vi "SMO.Activity.GetActivityManager.vi"(8 "error in (no error)":errorcluster, 11 "SMO.Activity":refnum<class "SMO.Activity.lvclass">) -> (0 "error out":errorcluster, 3 "SMO.Activity out":refnum<class "SMO.Activity.lvclass">)   [LabVIEW 2015, in "SMO.Activity.lvclass"]
uses:
  SMO.Activity.lvclass
  SMO.Activity.lvclass/SMO.Activity.ctl
panel:
  # "For instructions on how to use the JKI State Machine Objects, examples and video tutorials, visit:\nhttp://jki.net/state-machine-objects/\n\nJKI State Machine Objects™\nhttp://jki.net/state-machine-objects/\nCopyright (C) 2005-2015, JKI <info@jki.net>\nALL RIGHTS RESERVED"
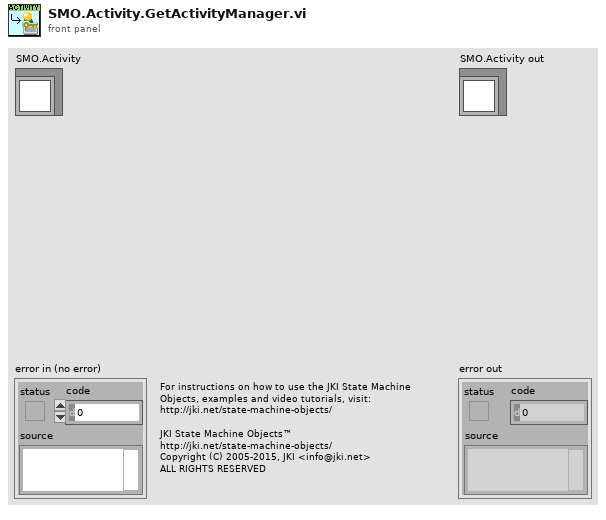
[diagram p1: front panel]
types:
  T1 = typedef "SMO.Activity.lvclass/PrivateData--Ref.ctl" = refnum<data-value>
  T2 = typedef "SMO.Activity.lvclass/PrivateData--Cluster.ctl" = cluster{"Public Events":T3, "Subpanel Ref":refnum<vi>, "UI State":T4}
  T3 = typedef "SMO.Activity.lvclass/PublicEvents--Cluster.ctl" = cluster{"UI State":refnum<user-event>}
  T4 = typedef "SMO.Activity.lvclass/SMO.UI_Embed State--enum.ctl" = enum16{"unknown", "Opened", "Embedded", "Closed"}
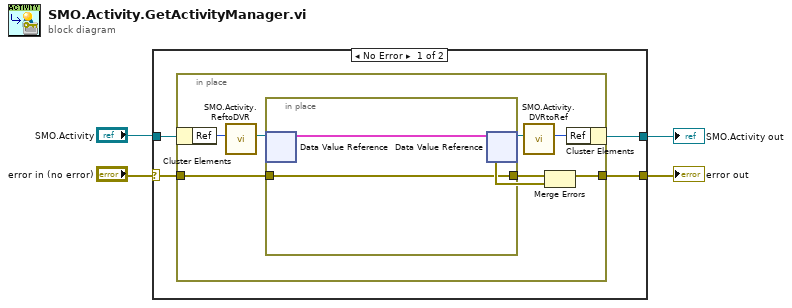
[diagram p0: block diagram]
diagram:
  n1 = case shown="No Error" "error in (no error)" {
    selector: "error in (no error)" -> [w7 w20]
    tunnel: [w6 w20] -> w1
    tunnel: [w5 w19] -> w3
    tunnel: "SMO.Activity" -> [w8 w19]
    frame No Error {
      n2 = in-place {
        in-place-border: w7 -> [w16]
        in-place-border: [w13] -> w6
        n3 = in-place-cluster #1(w8) -> ("Ref"=w10:u32)
        n4 = call "SMO.Activity.ReftoDVR.vi"("Ref"=w10) -> ("Ref"=w9:T1)  [unwired: 10 in]
        n5 = in-place {
          in-place-border: w16 -> [w18]
          in-place-border: [w18] -> w14
          n6 = in-place-dvr #2(w9) -> (w17:T2)  [unwired: 1 out]
          n7 = in-place-dvr #2(w17) -> (w12:T1, w15:errorcluster)
        }
        n8 = call "SMO.Activity.DVRtoRef.vi"("Ref"=w12) -> ("Ref"=w11:u32)  [unwired: 10 in]
        n9 = Merge Errors(w14, w15) -> (w13:errorcluster)
        n10 = in-place-cluster #1("Ref"=w11) -> (w5:refnum<class "SMO.Activity.lvclass">)
      }
    }
    frame Error {
    }
  }
  "error out" <- w1
  "SMO.Activity out" <- w3
